vi "Rig_Pict_Display_Pref.vi"(0 "Traverse Name":string) -> (1 "Roll Pitch Yaw ADAM Channels":string[](array[string]), 4 "Which Axis is vertical?":enum16{"X Axis", "Y Axis", "Z Axis"}(ring), 5 "Position Feedback System":T1, 6 "Plan View":T2, 7 "Side View":T2, 8 "Front View":T2)   [LabVIEW 2022 SP3]
uses:
  Pict_Plot_Axis.ctl
  Axis.ctl
  Controls/Position Feedback System.ctl
  Globals/Constants_global.vi
  Globals/Trav_pos_global.vi
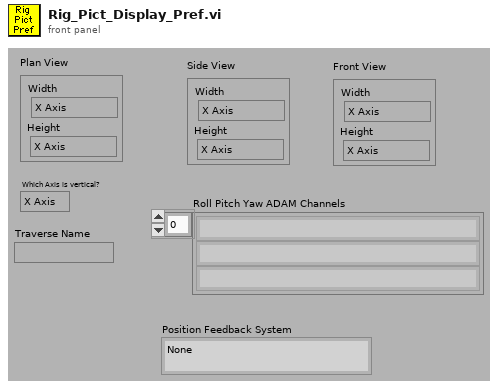
[diagram p1: front panel]
types:
  T1 = typedef "Position Feedback System.ctl" = enum16{"None", "OptiTrack"}
  T2 = typedef "Pict_Plot_Axis.ctl" = cluster{"Width":T3, "Height":T3}
  T3 = typedef "Axis.ctl" = enum16{"X Axis", "X Axis -ve", "Y Axis", "Y Axis -ve", "Z Axis", "Z Axis -ve"}
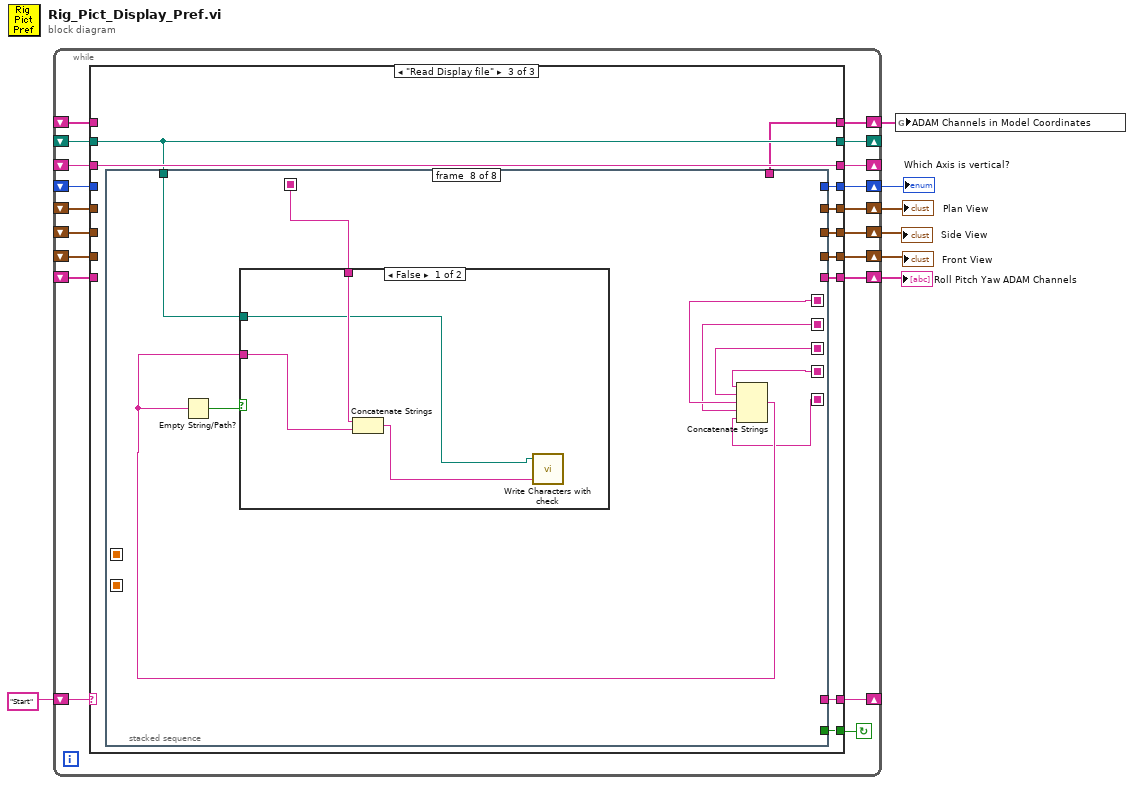
[diagram p0: block diagram]
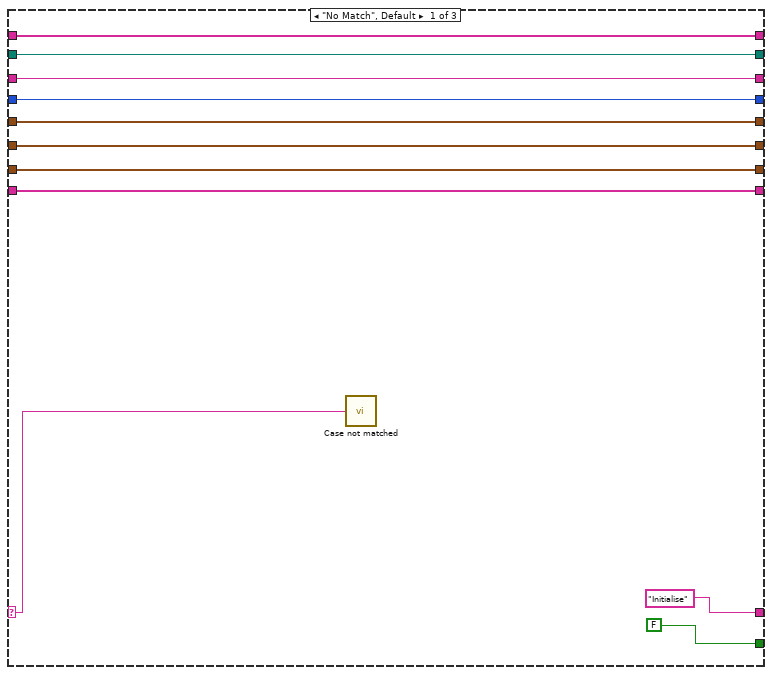
[diagram p2: hidden frame]
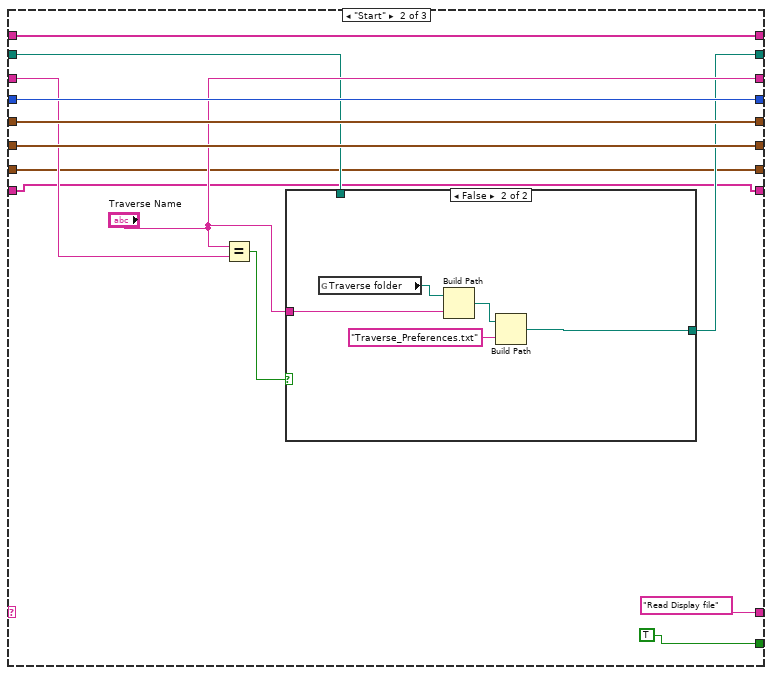
[diagram p3: hidden frame]
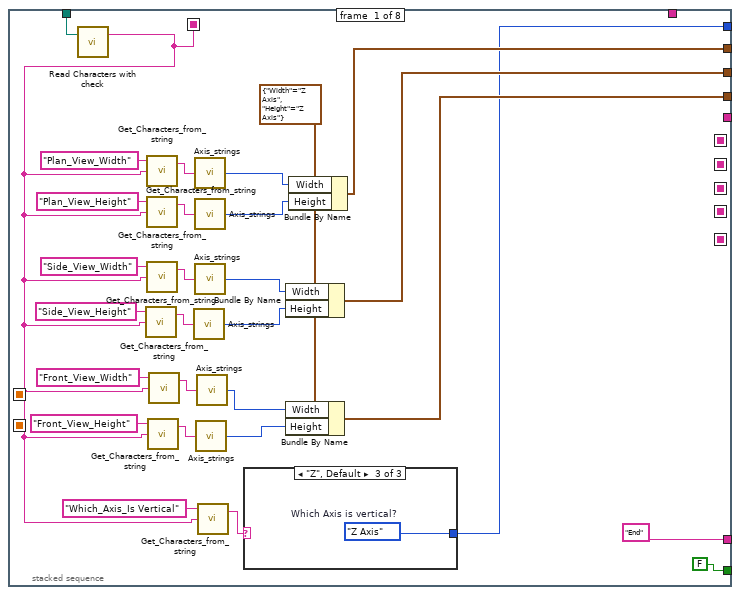
[diagram p5: hidden frame]
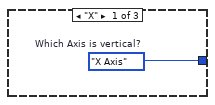
[diagram p6: hidden frame]
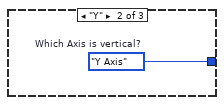
[diagram p7: hidden frame]
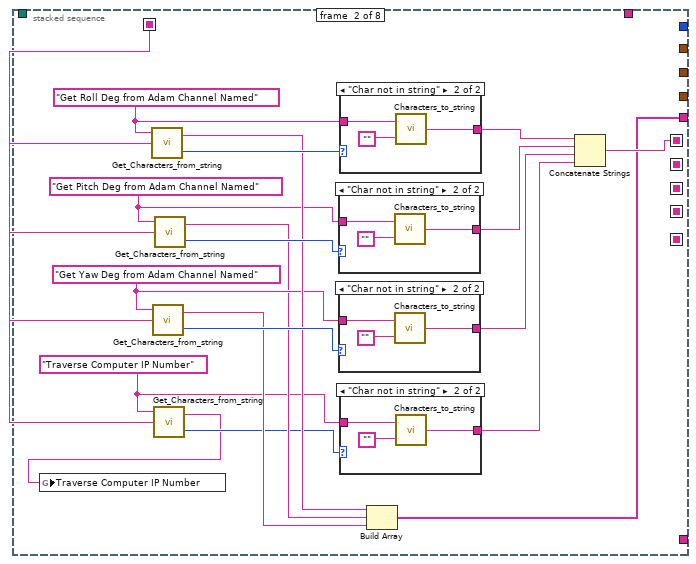
[diagram p8: hidden frame]
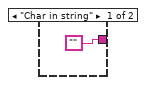
[diagram p9: hidden frame]
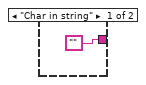
[diagram p10: hidden frame]
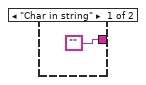
[diagram p11: hidden frame]
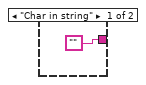
[diagram p12: hidden frame]
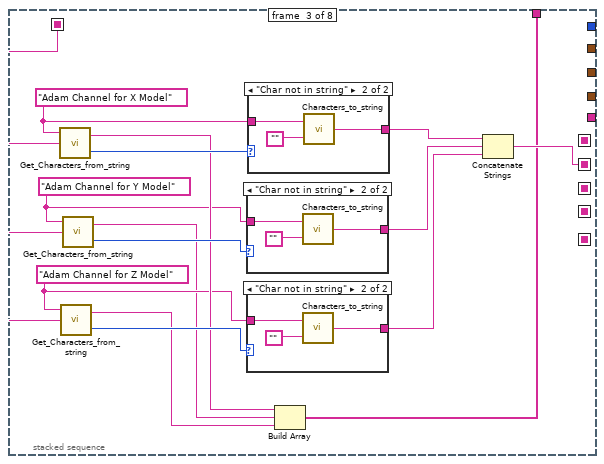
[diagram p13: hidden frame]
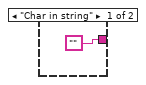
[diagram p14: hidden frame]
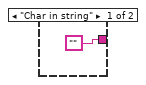
[diagram p15: hidden frame]
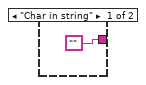
[diagram p16: hidden frame]
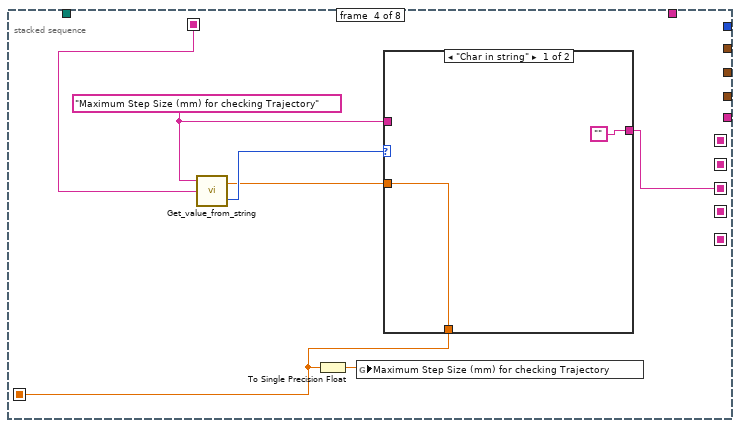
[diagram p17: hidden frame]
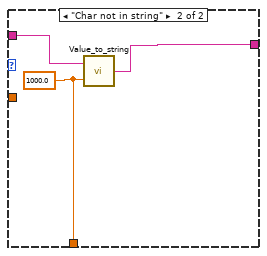
[diagram p18: hidden frame]
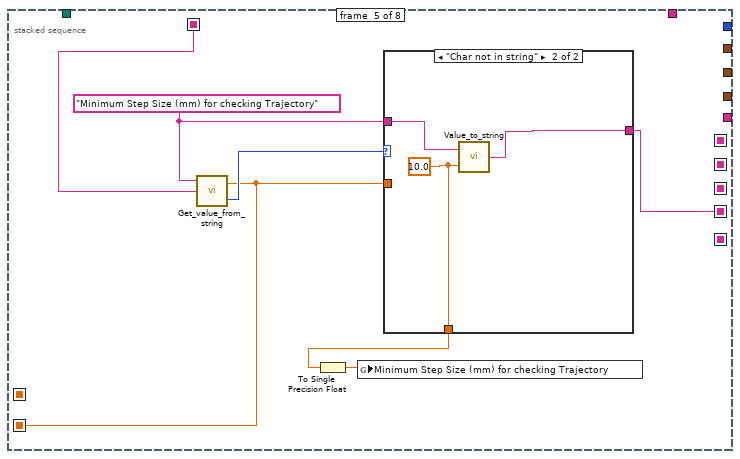
[diagram p19: hidden frame]
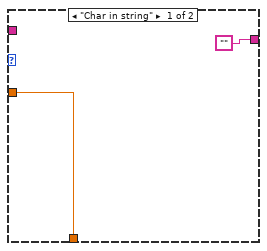
[diagram p20: hidden frame]
diagram:
  n1 = while {
    shift-left: "Start" -> [w24]
    shift-right: [w25] -> _
    shift-right: [w22] -> _
    shift-left: _ -> [w23]
    shift-right: [w16] -> w3
    shift-left: _ -> [w17]
    shift-right: [w19] -> w6
    shift-left: _ -> [w18]
    shift-right: [w20] -> w5
    shift-left: _ -> [w21]
    shift-right: [w15] -> _
    shift-left: _ -> [w14]
    shift-right: [w12] -> w4
    shift-left: _ -> [w13]
    shift-right: [w11] -> w2
    shift-left: _ -> [w10]
    shift-right: [w9] -> w1
    shift-left: _ -> [w8]
    stop <- w26 continue-if-true
    n2 = case shown="\"Read Display file\"" w24 {
      selector: w24 -> [w27 _ _]
      tunnel: [FALSE TRUE ("Modified?") w59] -> w26
      tunnel: ["Initialise" "Read Display file" w66] -> w25
      tunnel: w23 -> [w34 w46 w65]
      tunnel: [w34 "Traverse Name" w65] -> w22
      tunnel: w21 -> [w31 w49 _]
      tunnel: [w31 w49 w62] -> w20
      tunnel: [w32 w48 w63] -> w19
      tunnel: w18 -> [w32 w48 _]
      tunnel: w17 -> [w33 w47 _]
      tunnel: [w33 w47 w60] -> w16
      tunnel: [w35 w44 w64] -> w15
      tunnel: w14 -> [w35 w42 w64]
      tunnel: w13 -> [w30 w41 _]
      tunnel: [w30 w41 w61] -> w12
      tunnel: [w29 w40 w58] -> w11
      tunnel: w10 -> [w29 w40 _]
      tunnel: [w28 w38 w57] -> w9
      tunnel: w8 -> [w28 w38 _]
      frame "No Match", Default {
        n3 = call "Case not matched.vi"("Case Name not Matched"=w27) -> ()
      }
      frame "Start" {
        n4 = Equal?(x="Traverse Name", y=w46) -> (x = y?=w43:bool)
        n5 = case shown="False" w43 {
          tunnel: "Traverse Name" -> [_ w55]
          tunnel: [w51 w52] -> w44
          tunnel: w42 -> [w51 _]
          frame True {
          }
          frame False {
            n6 = global read "Constants_global.vi" "Traverse folder"() -> (w56:path)
            n7 = Build Path(base path=w56, name or relative path=w55) -> (appended path=w54:path)
            n8 = Build Path(base path=w54, name or relative path="Traverse_Preferences.txt") -> (appended path=w52:path)
          }
        }
      }
      frame "Read Display file" {
        n9 = stacked-sequence {
          seq-local: [w67 _ _ _ _ _ _ _] -> [_ w102 w136 w165 w177 w192 _ w213]
          seq-local: [_ w105 _ _ _ _ _ _] -> [_ _ _ _ _ _ _ w217]
          seq-local: [_ _ _ w164 _ _ _ _] -> [_ _ _ _ _ _ _ w214]
          seq-local: [_ _ w135 _ _ _ _ _] -> [_ _ _ _ _ _ _ w216]
          seq-local: [_ _ _ _ w174 _ _ _] -> [_ _ _ _ _ _ _ w211]
          seq-local: [_ _ _ w161 _ _ _ _] -> [_ _ _ _ _ _ w204 _]
          seq-local: [_ _ _ _ w173 _ _ _] -> [_ _ _ _ _ _ w203 _]
          seq-local: [_ _ _ _ _ w189 _ _] -> [_ _ _ _ _ _ _ w210]
          tunnel: ["End" _ _ _ _ _ _ _] -> w66
          tunnel: w64 -> [w68 _ _ _ _ _ w201 w218]
          tunnel: [w75 _ _ _ _ _ _ _] -> w63
          tunnel: [w74 _ _ _ _ _ _ _] -> w62
          tunnel: [w73 _ _ _ _ _ _ _] -> w61
          tunnel: [w70 _ _ _ _ _ _ _] -> w60
          tunnel: [FALSE ("Modified?") _ _ _ _ _ _ _] -> w59
          tunnel: [_ w104 _ _ _ _ _ _] -> w58
          tunnel: [_ _ w134 _ _ _ _ _] -> w57
          frame #0 {
            w80 = T2 {"Width"=enum."Z Axis", "Height"=enum."Z Axis"} ("Plot Axis")
            n10 = call "Read Characters with check.vi"("file (use dialog)"=w68) -> ("Read String"=w67:string)  [unwired: 1 in, 1 out]
            n11 = call "Get_Characters_from_string.vi"("Input string"=w67, "Variable name"="Side_View_Height") -> ("Value"=w88:string)  [unwired: 1 in, 1 out]
            n12 = call "Get_Characters_from_string.vi"("Input string"=w67, "Variable name"="Plan_View_Width") -> ("Value"=w93:string)  [unwired: 1 in, 1 out]
            n13 = call "Get_Characters_from_string.vi"("Input string"=w67, "Variable name"="Plan_View_Height") -> ("Value"=w92:string)  [unwired: 1 in, 1 out]
            n14 = call "Get_Characters_from_string.vi"("Input string"=w67, "Variable name"="Side_View_Width") -> ("Value"=w89:string)  [unwired: 1 in, 1 out]
            n15 = call "Get_Characters_from_string.vi"("Input string"=w67, "Variable name"="Front_View_Height") -> ("Value"=w84:string)  [unwired: 1 in, 1 out]
            n16 = call "Get_Characters_from_string.vi"("Input string"=w67, "Variable name"="Front_View_Width") -> ("Value"=w85:string)  [unwired: 1 in, 1 out]
            n17 = call "Axis_strings.vi"("String"=w88) -> ("Enum"=w76:T3)
            n18 = call "Axis_strings.vi"("String"=w93) -> ("Enum"=w79:T3)
            n19 = call "Axis_strings.vi"("String"=w92) -> ("Enum"=w78:T3)
            n20 = call "Axis_strings.vi"("String"=w89) -> ("Enum"=w77:T3)
            n21 = call "Axis_strings.vi"("String"=w84) -> ("Enum"=w81:T3)
            n22 = call "Axis_strings.vi"("String"=w85) -> ("Enum"=w82:T3)
            n23 = call "Get_Characters_from_string.vi"("Input string"=w67, "Variable name"="Which_Axis_Is Vertical") -> ("Value"=w71:string)  [unwired: 1 in, 1 out]
            n24 = case shown="\"Z\", Default" w71 {
              tunnel: [w96 w97 w98] -> w70
              frame "X" {
                w96 = enum16{"X Axis", "Y Axis", "Z Axis"}."X Axis"  # Which Axis is vertical?
              }
              frame "Y" {
                w97 = enum16{"X Axis", "Y Axis", "Z Axis"}."Y Axis"  # Which Axis is vertical?
              }
              frame "Z", Default {
                w98 = enum16{"X Axis", "Y Axis", "Z Axis"}."Z Axis"  # Which Axis is vertical?
              }
            }
            n25 = Bundle By Name(cluster=w80, "Width"=w77, "Height"=w76) -> (w74:T2)
            n26 = Bundle By Name(cluster=w80, "Width"=w82, "Height"=w81) -> (w73:T2)
            n27 = Bundle By Name(cluster=w80, "Width"=w79, "Height"=w78) -> (w75:T2)
          }
          frame #1 {
            w101 = "Traverse Computer IP Number" ("Variable name")
            w108 = "Get Yaw Deg from Adam Channel Named" ("Variable name")
            w109 = "Get Pitch Deg from Adam Channel Named" ("Variable name")
            w116 = "Get Roll Deg from Adam Channel Named" ("Variable name")
            n28 = call "Get_Characters_from_string.vi"("Input string"=w102, "Variable name"=w116) -> ("Status"=w117:enum16{"Char in string", "Char not in string"}, "Value"=w110:string)  [unwired: 1 in]
            n29 = call "Get_Characters_from_string.vi"("Input string"=w102, "Variable name"=w108) -> ("Status"=w113:enum16{"Char in string", "Char not in string"}, "Value"=w106:string)  [unwired: 1 in]
            n30 = call "Get_Characters_from_string.vi"("Input string"=w102, "Variable name"=w101) -> ("Status"=w103:enum16{"Char in string", "Char not in string"}, "Value"=w99:string)  [unwired: 1 in]
            n31 = global write "Trav_pos_global.vi" "Traverse Computer IP Number"(w99) -> ()
            n32 = call "Get_Characters_from_string.vi"("Input string"=w102, "Variable name"=w109) -> ("Status"=w114:enum16{"Char in string", "Char not in string"}, "Value"=w107:string)  [unwired: 1 in]
            n33 = case shown="\"Char not in string\"" w114 {
              tunnel: w109 -> [_ w129]
              tunnel: ["" w127] -> w112
              frame "Char in string" {
              }
              frame "Char not in string" {
                n34 = call "Characters_to_string.vi"("Characters to write"="", "Label for characters"=w129) -> ("Output string"=w127:string)  [unwired: 1 in]
              }
            }
            n35 = case shown="\"Char not in string\"" w113 {
              tunnel: w108 -> [_ w125]
              tunnel: ["" w123] -> w111
              frame "Char in string" {
              }
              frame "Char not in string" {
                n36 = call "Characters_to_string.vi"("Characters to write"="", "Label for characters"=w125) -> ("Output string"=w123:string)  [unwired: 1 in]
              }
            }
            n37 = case shown="\"Char not in string\"" w117 {
              tunnel: w116 -> [_ w133]
              tunnel: ["" w131] -> w115
              frame "Char in string" {
              }
              frame "Char not in string" {
                n38 = call "Characters_to_string.vi"("Characters to write"="", "Label for characters"=w133) -> ("Output string"=w131:string)  [unwired: 1 in]
              }
            }
            n39 = case shown="\"Char not in string\"" w103 {
              tunnel: w101 -> [_ w121]
              tunnel: ["" w119] -> w100
              frame "Char in string" {
              }
              frame "Char not in string" {
                n40 = call "Characters_to_string.vi"("Characters to write"="", "Label for characters"=w121) -> ("Output string"=w119:string)  [unwired: 1 in]
              }
            }
            n41 = Build Array(w110, w107, w106) -> (w104:string[])
            n42 = Concatenate Strings(w115, w112, w111, w100) -> (w105:string)
          }
          frame #2 {
            w139 = "Adam Channel for Z Model" ("Variable name")
            w140 = "Adam Channel for Y Model" ("Variable name")
            w147 = "Adam Channel for X Model" ("Variable name")
            n43 = call "Get_Characters_from_string.vi"("Input string"=w136, "Variable name"=w147) -> ("Status"=w148:enum16{"Char in string", "Char not in string"}, "Value"=w141:string)  [unwired: 1 in]
            n44 = call "Get_Characters_from_string.vi"("Input string"=w136, "Variable name"=w139) -> ("Status"=w144:enum16{"Char in string", "Char not in string"}, "Value"=w137:string)  [unwired: 1 in]
            n45 = call "Get_Characters_from_string.vi"("Input string"=w136, "Variable name"=w140) -> ("Status"=w145:enum16{"Char in string", "Char not in string"}, "Value"=w138:string)  [unwired: 1 in]
            n46 = case shown="\"Char not in string\"" w145 {
              tunnel: w140 -> [_ w156]
              tunnel: ["" w154] -> w143
              frame "Char in string" {
              }
              frame "Char not in string" {
                n47 = call "Characters_to_string.vi"("Characters to write"="", "Label for characters"=w156) -> ("Output string"=w154:string)  [unwired: 1 in]
              }
            }
            n48 = case shown="\"Char not in string\"" w144 {
              tunnel: w139 -> [_ w152]
              tunnel: ["" w150] -> w142
              frame "Char in string" {
              }
              frame "Char not in string" {
                n49 = call "Characters_to_string.vi"("Characters to write"="", "Label for characters"=w152) -> ("Output string"=w150:string)  [unwired: 1 in]
              }
            }
            n50 = case shown="\"Char not in string\"" w148 {
              tunnel: w147 -> [_ w160]
              tunnel: ["" w158] -> w146
              frame "Char in string" {
              }
              frame "Char not in string" {
                n51 = call "Characters_to_string.vi"("Characters to write"="", "Label for characters"=w160) -> ("Output string"=w158:string)  [unwired: 1 in]
              }
            }
            n52 = Build Array(w141, w138, w137) -> (w134:string[])
            n53 = Concatenate Strings(w146, w143, w142) -> (w135:string)
          }
          frame #3 {
            w167 = "Maximum Step Size (mm) for checking Trajectory" ("Variable name")
            n54 = call "Get_value_from_string.vi"("Input string"=w165, "Variable name"=w167) -> ("Status"=w166:enum16{"Char in string", "Char not in string"}, "Value"=w163:dbl)  [unwired: 1 in]
            n55 = case shown="\"Char in string\"" w166 {
              tunnel: w167 -> [_ w172]
              tunnel: ["" w170] -> w164
              tunnel: [w169 w171] -> w161
              tunnel: w163 -> [w169 _]
              frame "Char in string" {
              }
              frame "Char not in string" {
                w171 = 1000.0 ("Value")
                n56 = call "Value_to_string.vi"("Value"=w171, "Label for value"=w172) -> ("Output string"=w170:string)  [unwired: 1 in]
              }
            }
            n57 = To Single Precision Float(number=w161) -> (single precision float=w162:sgl)
            n58 = global write "Trav_pos_global.vi" "Maximum Step Size (mm) for checking Trajectory"(w162) -> ()
          }
          frame #4 {
            w179 = "Minimum Step Size (mm) for checking Trajectory" ("Variable name")
            n59 = call "Get_value_from_string.vi"("Input string"=w177, "Variable name"=w179) -> ("Status"=w178:enum16{"Char in string", "Char not in string"}, "Value"=w173:dbl)  [unwired: 1 in]
            n60 = case shown="\"Char not in string\"" w178 {
              tunnel: w179 -> [_ w184]
              tunnel: ["" w182] -> w174
              tunnel: [w181 w183] -> w176
              tunnel: w173 -> [w181 _]
              frame "Char in string" {
              }
              frame "Char not in string" {
                w183 = 10.0 ("Value")
                n61 = call "Value_to_string.vi"("Value"=w183, "Label for value"=w184) -> ("Output string"=w182:string)  [unwired: 1 in]
              }
            }
            n62 = To Single Precision Float(number=w176) -> (single precision float=w175:sgl)
            n63 = global write "Trav_pos_global.vi" "Minimum Step Size (mm) for checking Trajectory"(w175) -> ()
          }
          frame #5 {
            w193 = "Position Feedback System" ("Variable name")
            n64 = call "Get_Characters_from_string.vi"("Input string"=w192, "Variable name"=w193) -> ("Status"=w191:enum16{"Char in string", "Char not in string"}, "Value"=w190:string)  [unwired: 1 in]
            n65 = case shown="\"Char in string\"" w191 {
              tunnel: w193 -> [_ w200]
              tunnel: ["" w199] -> w189
              tunnel: [w197 w198] -> w188
              tunnel: w190 -> [w197 _]
              frame "Char in string" {
              }
              frame "Char not in string" {
                w198 = ""
                n66 = call "Characters_to_string.vi"("Characters to write"=w198, "Label for characters"=w200) -> ("Output string"=w199:string)  [unwired: 1 in]
              }
            }
            n67 = String Subset(string=w188, length (rest)=4 ("length (rest)")) -> (substring=w186:string)  [unwired: 1 in]
            n68 = case shown="Default" w186 {
              tunnel: [Position_Feedback_System."None" ("Enum") Position_Feedback_System."OptiTrack" ("Enum")] -> w185
              frame Default {
              }
              frame "Opti" {
              }
            }
            "Position Feedback System" <- w185
          }
          frame #6 {
            n69 = Greater?(x=w204, y=w203) -> (0:w202:bool)
            n70 = case shown="False" w202 {
              tunnel: w201 -> [w209 _]
              frame False {
                n71 = Format Into String(format string="Minimum Step Size (mm) for checking Trajectory must be less than the maximum see file\n%s", w209) -> (resulting string=w207:string)  [unwired: 2 in, 1 out]
                n72 = One Button Dialog(message=w207, button name ("OK")="Stop") -> (true=w205:bool)
                n73 = Stop(stop? (T)=w205) -> ()
              }
              frame True {
              }
            }
          }
          frame #7 {
            n74 = Concatenate Strings(w211, w214, w217, w216, w210) -> (w215:string)
            n75 = Empty String/Path?(string/path=w215) -> (empty?=w212:bool)
            n76 = case shown="False" w212 {
              tunnel: w215 -> [w221 _]
              tunnel: w218 -> [w220 _]
              tunnel: w213 -> [w222 _]
              frame False {
                n77 = Concatenate Strings(w222, w221) -> (w219:string)
                n78 = call "Write Characters with check.vi"("String to Write"=w219, "file (use dialog)"=w220) -> ()  [unwired: 2 in, 1 out]
              }
              frame True {
              }
            }
          }
        }
      }
    }
  }
  "Plan View" <- w6
  "Side View" <- w5
  "Front View" <- w4
  "Which Axis is vertical?" <- w3
  "Roll Pitch Yaw ADAM Channels" <- w2
  n79 = global write "Trav_pos_global.vi" "ADAM Channels in Model Coordinates"(w1) -> ()
